vi "ExSubReadFileSPE.vi"(2 "error in (no error)":errorcluster, 3 "Frame Number":u32, 4 "File Name":string) -> (0 "error out":errorcluster, 1 "Image Handle":u32)   [LabVIEW 2010]
panel:
  # "ExSubReadFileSPE:\nThis SubVI opens a file\nand reads the frame \nnumber supplied, it then\ncloses the file and returns\nhandle to frame data \nread."
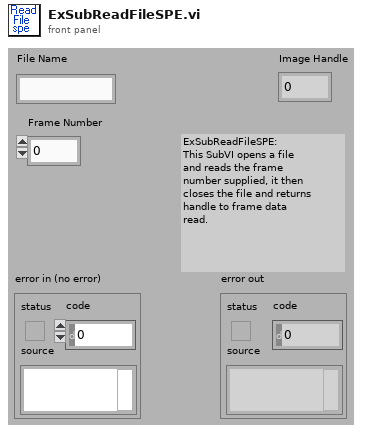
[diagram p1: front panel]
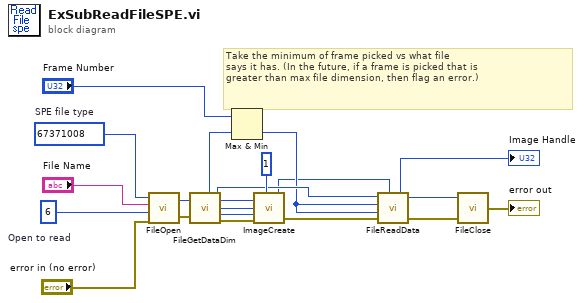
[diagram p0: block diagram]
diagram:
  w12 = 6  # Open to read
  w14 = u32 67371008  # SPE file type
  # "Take the minimum of frame picked vs what file\nsays it has. (In the future, if a frame is picked that is\ngreater than max file dimension, then flag an error.)"
  n1 = call <userlib>:"FileOpen.vi"("error in"="error in (no error)", "File Operations"=w12, "FileName"="File Name", "File Type"=w14) -> ("error out"=w20:errorcluster, "File Handle"=w21:u32)
  n2 = call <userlib>:"FileGetDataDim.vi"("File Handle"=w21, "error in"=w20) -> ("Number of Frames"=w10:u32, "Data Type"=w18:u32, "File Handle"=w8:u32, "X dim"=w15:u32, "Y dim"=w17:u32, "error out"=w19:errorcluster)
  n3 = Max & Min(x="Frame Number", y=w10) -> (min(x,y)=w7:u32)  [unwired: 1 out]
  n4 = call <userlib>:"ImageCreate.vi"("X dimension"=w15, "Y dimension"=w17, "Data Type"=w18, "error in"=w19, "Number Of Frames"=1) -> ("Image Handle"=w5:u32, "error out"=w6:errorcluster)
  n5 = call <userlib>:"FileReadData.vi"("File Handle"=w8, "Start Frame"=w7, "End Frame"=w7, "error in"=w6, "Image Handle"=w5) -> ("File Handle"=w4:u32, "Image Handle"=→"Image Handle":u32, "error out"=w3:errorcluster)
  n6 = call <userlib>:"FileClose.vi"("error in"=w3, "File Handle"=w4) -> ("error out"=→"error out":errorcluster)
